vi "GetStepData.vi"(8 "error in (no error)":errorcluster, 11 "Index":T1) -> (0 "error out":errorcluster, 2 "Valid?":bool, 3 "Data":variant)   [LabVIEW 2016, in "SeqProcessor.lvlib"]
uses:
  SeqProcessor.lvlib
  controls/StepIndex.ctl
  controls/NormalStep.ctl
  controls/StepAction.ctl
  controls/StepResult.ctl
  controls/StepStatus.ctl
  controls/JumpStep.ctl
  controls/ConditionalStep.ctl
  controls/ParallelStep.ctl
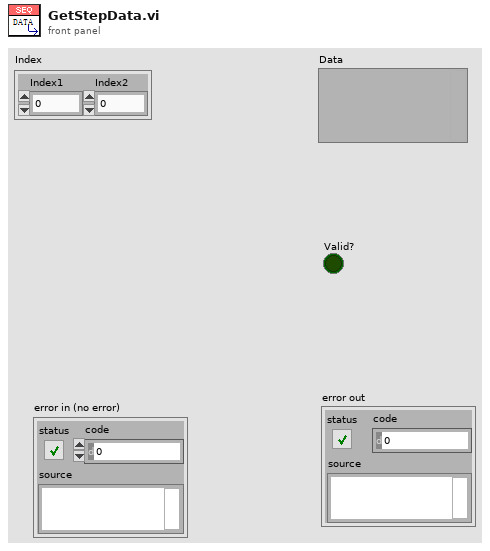
[diagram p1: front panel]
types:
  T1 = typedef "SeqProcessor.lvlib/StepIndex.ctl" = cluster{"Index1":u32, "Index2":u32}
  T2 = typedef "SeqProcessor.lvlib/Step.ctl" = cluster{"Type":T3, "Step":variant}
  T3 = typedef "SeqProcessor.lvlib/StepType.ctl" = enum16{"Normal", "Parallel", "Conditional", "Jump"}
  T4 = typedef "SeqProcessor.lvlib/NormalStep.ctl" = cluster{"Action":T5, "Result":T6}
  T5 = typedef "SeqProcessor.lvlib/StepAction.ctl" = cluster{"Action":string, "Process":string, "Data":variant, "Condition":variant}
  T6 = typedef "SeqProcessor.lvlib/StepResult.ctl" = cluster{"Status":T7, "Message":string, "Data":variant}
  T7 = typedef "SeqProcessor.lvlib/StepStatus.ctl" = enum16{"Undone", "Finish", "Error"}
  T8 = typedef "SeqProcessor.lvlib/JumpStep.ctl" = cluster{"Action":T5, "Jump":i32, "Result":T6}
  T9 = typedef "SeqProcessor.lvlib/ConditionalStep.ctl" = cluster{"Action":T5, "Result":T6}
  T10 = typedef "SeqProcessor.lvlib/ParallelStep.ctl" = T4[]
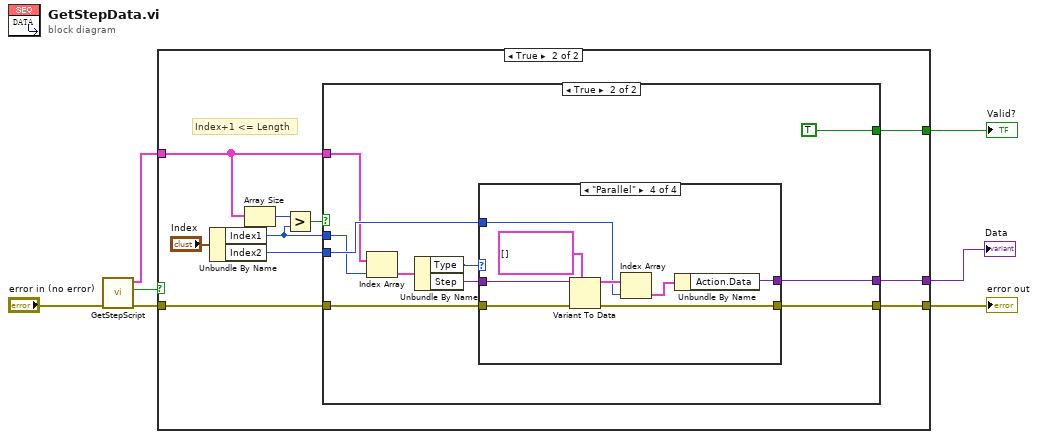
[diagram p0: block diagram]
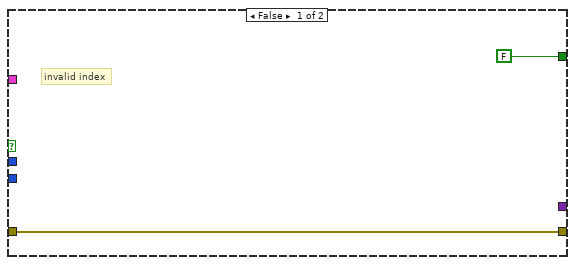
[diagram p3: hidden frame]
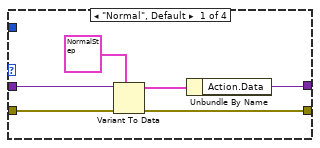
[diagram p4: hidden frame]
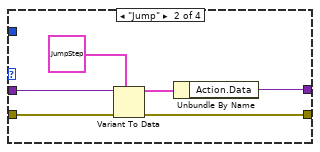
[diagram p5: hidden frame]
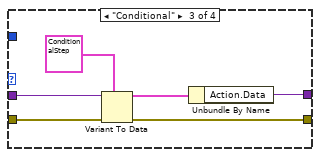
[diagram p6: hidden frame]
diagram:
  n1 = call "GetStepScript.vi"("error in (no error)"="error in (no error)") -> ("error out"=w5:errorcluster, "found"=w6:bool, "StepScript"=w4:T2[])  [unwired: 8 in]
  n2 = case shown="True" w6 {
    selector: w6 -> [w8 _]
    tunnel: w5 -> [w9 w19]
    tunnel: w4 -> [_ w17]
    tunnel: [w9 w12] -> w3
    tunnel: [w8 w11] -> w2
    tunnel: [_ w10] -> w1
    frame False {
    }
    frame True {
      # "Index+1 <= Length"
      n3 = Unbundle By Name("Index") -> ("Index1"=w15:u32, "Index2"=w13:u32)
      n4 = Array Size(array=w17) -> (size(s)=w16:i32)
      n5 = Greater?(x=w16, y=w15) -> (0:w14:bool)
      n6 = case shown="True" w14 {
        tunnel: w19 -> [w21 w29]
        tunnel: w17 -> [_ w27]
        tunnel: w15 -> [_ w25]
        tunnel: w13 -> [_ w28]
        tunnel: [w21 w23] -> w12
        tunnel: [FALSE TRUE] -> w11
        tunnel: [_ w22] -> w10
        frame False {
          # "invalid index"
        }
        frame True {
          n7 = Index Array(array=w27, index=w25) -> (element=w26:T2)
          n8 = Unbundle By Name(w26) -> ("Type"=w31:T3, "Step"=w30:variant)
          n9 = case shown="\"Parallel\"" w31 {
            tunnel: w30 -> [w37 w43 w49 w57]
            tunnel: w29 -> [w35 w42 w48 w56]
            tunnel: [w34 w41 w47 w55] -> w23
            tunnel: w28 -> [_ _ _ w52]
            tunnel: [w32 w38 w44 w50] -> w22
            frame "Normal", Default {
              n10 = Variant To Data(error in=w35, type=T4 {"Action"={"Action"="", "Process"="", "Data"=variant, "Condition"=variant(bool FALSE)}, "Result"={"Status"=enum."Undone", "Message"="", "Data"=variant}} ("NormalStep"), Variant=w37) -> (data=w33:T4, error out=w34:errorcluster)
              n11 = Unbundle By Name(w33) -> ("Action.Data"=w32:variant)
            }
            frame "Jump" {
              n12 = Variant To Data(error in=w42, type=T8 {"Action"={"Action"="", "Process"="", "Data"=variant, "Condition"=variant(bool FALSE)}, "Jump"=0, "Result"={"Status"=enum."Undone", "Message"="", "Data"=variant}} ("JumplStep"), Variant=w43) -> (data=w39:T8, error out=w41:errorcluster)
              n13 = Unbundle By Name(w39) -> ("Action.Data"=w38:variant)
            }
            frame "Conditional" {
              n14 = Variant To Data(error in=w48, type=T9 {"Action"={"Action"="", "Process"="", "Data"=variant, "Condition"=variant(bool FALSE)}, "Result"={"Status"=enum."Undone", "Message"="", "Data"=variant}} ("ConditionlStep"), Variant=w49) -> (data=w45:T9, error out=w47:errorcluster)
              n15 = Unbundle By Name(w45) -> ("Action.Data"=w44:variant)
            }
            frame "Parallel" {
              n16 = Variant To Data(error in=w56, type=T10 [] ("ParallelStep"), Variant=w57) -> (data=w53:T10, error out=w55:errorcluster)
              n17 = Index Array(array=w53, index=w52) -> (element=w51:T4)
              n18 = Unbundle By Name(w51) -> ("Action.Data"=w50:variant)
            }
          }
        }
      }
    }
  }
  "error out" <- w3
  "Valid?" <- w2
  "Data" <- w1
